vi "Write Data to Output File.vi"(5 "Pump Enable":string, 6 "Requested RPM":string, 7 "Pump PWM":string, 8 "Error In":errorcluster, 9 "Temperature":string, 10 "RPM":string, 11 "Output File":path) -> (0 "Error Out":errorcluster)   [LabVIEW 2017]
doc: "<b>Description</b>\nThis VI writes the run data into a csv file.\n\n<b>Inputs</b>\nOutput File: The file where the data will get written to. If the file already exists, data will be appended, not overwritten.\nRPM: The RPM measurement to record.\nTemperature: The temperature measurement to record.\nPump PWM: The pump PWM setting to record.\nPump Enable: The pump enable setting to record.\nRequested RPM: The Requested RPM setting to record."
uses:
  <vilib>/Utility/file.llb/Write Delimited Spreadsheet (string).vi
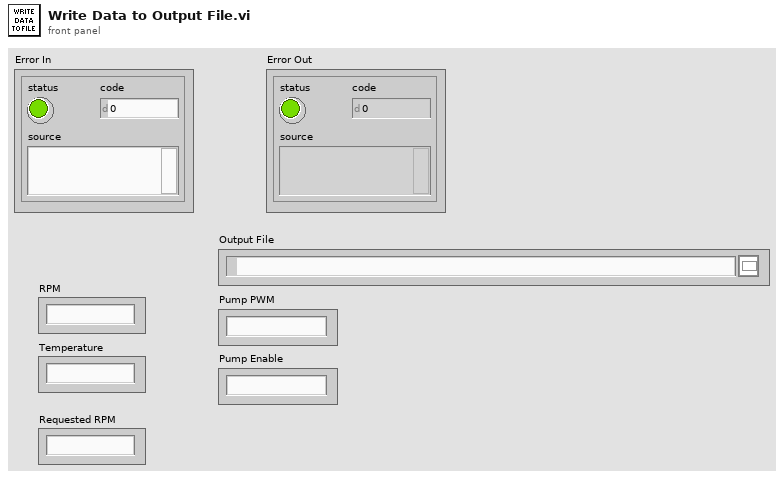
[diagram p1: front panel]
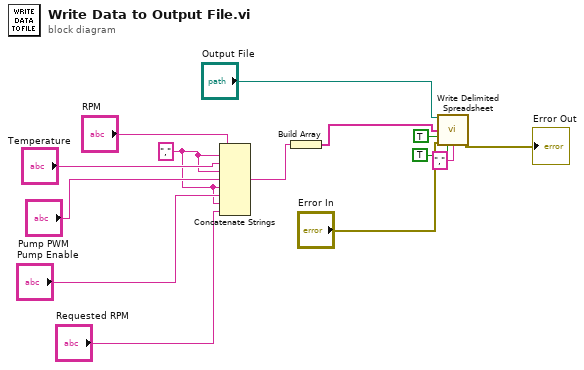
[diagram p0: block diagram]
diagram:
  w2 = "," ("string")
  n1 = Concatenate Strings("RPM", w2, "Temperature", w2, "Pump PWM", w2, "Pump Enable", w2, "Requested RPM") -> (w11:string)
  n2 = Build Array(w11) -> (w10:string[])
  n3 = call-poly <vilib>:"Write Delimited Spreadsheet.vi"("file path (dialog if empty)"="Output File", "1D data"=w10, "append to file? (new file:F)"=TRUE, "error in (no error)"="Error In", "transpose? (no:F)"=TRUE, "delimiter (\\t)"="," ("delimiter (\\t)")) -> ("error out"=→"Error Out":errorcluster)  [unwired: 8 in, 1 out]
